vi "write all Variants.vi"(8 "error in":errorcluster, 10 "values":variant[](array[variant]), 11 "data table in":T1) -> (0 "error out":errorcluster, 3 "data table out":T1)   [LabVIEW 2013, in "data bus values.lvlib"]
doc: "Replaces the entire set of values in the data table. If the size of the provided array does not match the array stored in the table, an error is thrown."
uses:
  data bus values.lvlib
  data table.ctl
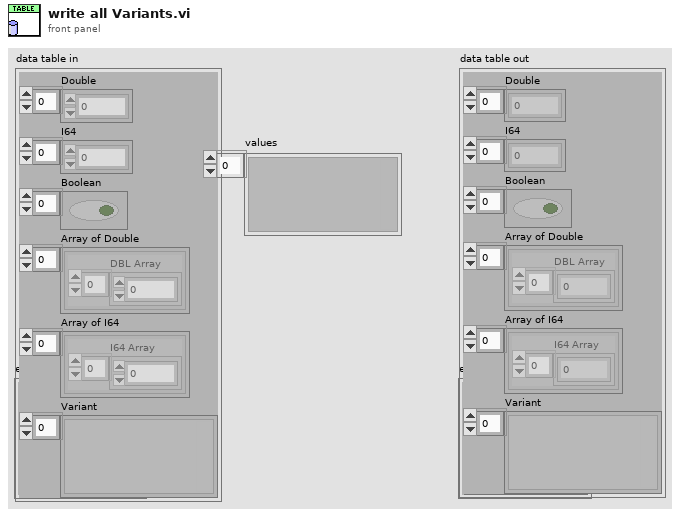
[diagram p1: front panel]
types:
  T1 = typedef "data bus values.lvlib/data table.ctl" = cluster{"Double":dbl[], "I64":i64[], "Boolean":bool[], "Array of Double":cluster{"DBL Array":dbl[]}[], "Array of I64":cluster{"I64 Array":i64[]}[], "Variant":variant[]}
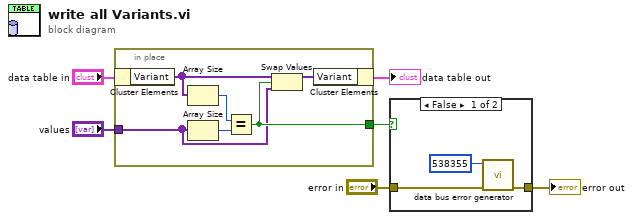
[diagram p0: block diagram]
diagram:
  n1 = in-place {
    in-place-border: [w8] -> w4
    in-place-border: "values" -> [w7]
    n2 = in-place-cluster #1("data table in") -> ("Variant"=w10:variant[])
    n3 = Array Size(array=w10) -> (size(s)=w12:i32)
    n4 = Array Size(array=w7) -> (size(s)=w11:i32)
    n5 = Equal?(x=w12, y=w11) -> (x = y?=w8:bool)
    n6 = Swap Values(12:w10, 13:w8, 14:w7) -> (1:w9:variant[])  [unwired: 1 out]
    n7 = in-place-cluster #1("Variant"=w9) -> (→"data table out":T1)
  }
  n8 = case shown="False" w4 {
    tunnel: [w15 w16] -> w3
    tunnel: "error in" -> [w14 w16]
    frame False {
      n9 = call "data bus error generator.vi"("error in"=w14, "error code (0)"=538355) -> ("error out"=w15:errorcluster)  [unwired: 7 in]
    }
    frame True {
    }
  }
  "error out" <- w3
